vi "test_dragon_file--move_version_to_subtable.vi"(8 "error in (no error)":errorcluster) -> (0 "error out":errorcluster)   [LabVIEW 2020]
uses:
  2bb1123c-6ef6-469c-ba61-7f462a8b3992.vi
  2bb1123c-6ef6-469c-ba61-7f462a8b3992.vi/4178f046-9af6-4db4-9405-99552d650b27.vi
  2bb1123c-6ef6-469c-ba61-7f462a8b3992.vi/504846f3-46c1-483c-ab2c-e4b1da560c38.vi
  toml/write_subtable_key_string.vi
  toml/toml.lvclass
  <vilib>/addons/_JKI Toolkits/Caraya/classes/Assert/Assert.lvclass
  <vilib>/addons/_JKI Toolkits/Caraya/classes/Test/Test.lvclass
panel:
  out "toml_string":string
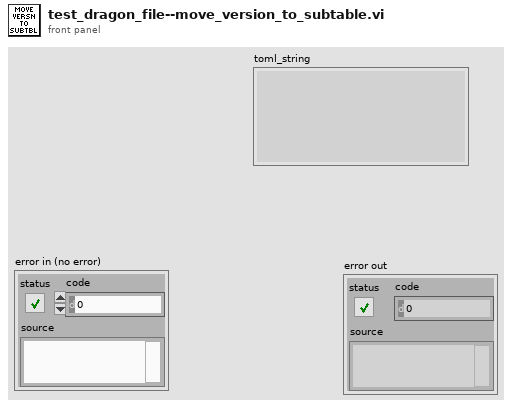
[diagram p1: front panel]
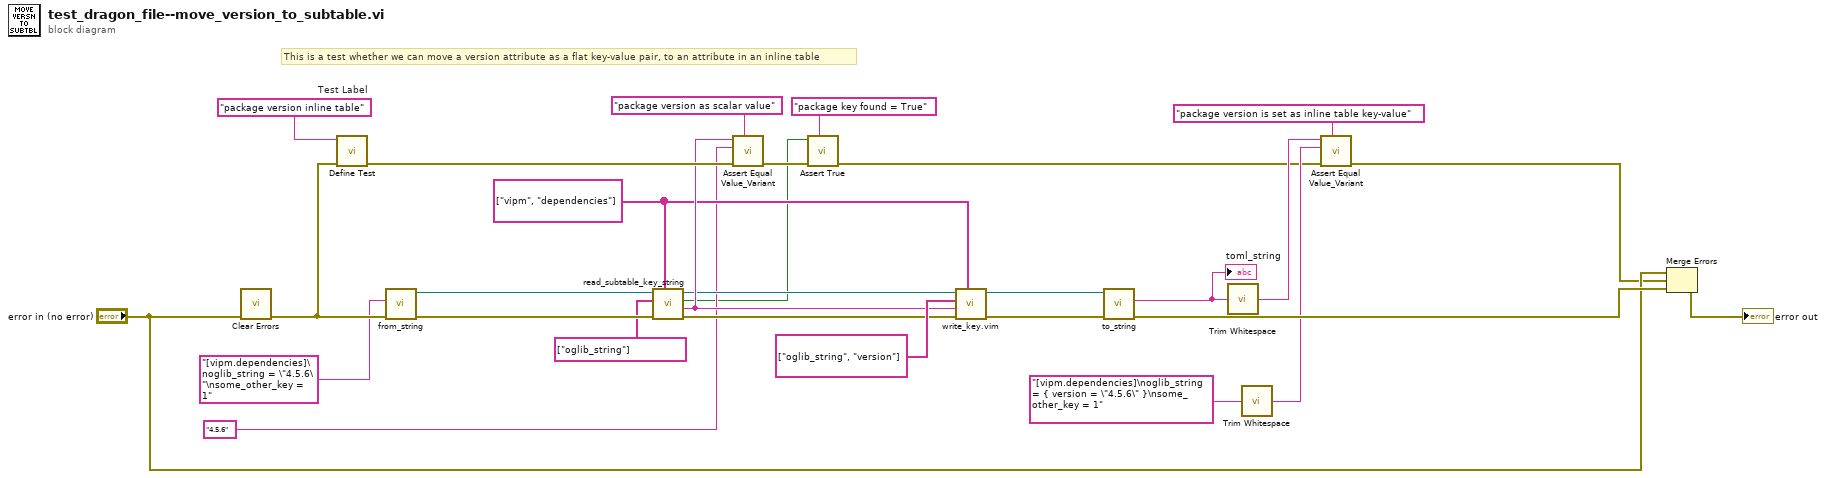
[diagram p0: block diagram]
diagram:
  w16 = string[] ["vipm", "dependencies"]
  w27 = "package version inline table"  # Test Label
  # "This is a test whether we can move a version attribute as a flat key-value pair, to an attribute in an inline table"
  n1 = call <vilib>:"Clear Errors.vi"("error in (no error)"="error in (no error)") -> ("error out"=w14:errorcluster)  [unwired: 5 in, 1 out]
  n2 = call <vilib>:"Define Test.vi"("error in (no error)"=w14, "Label (VI Title)"=w27) -> ("error out"=w28:errorcluster)  [unwired: 9 in]
  n3 = call "from_string.vi"("error in (no error)"=w14, "toml"="[vipm.dependencies]\noglib_string = \"4.5.6\"\nsome_other_key = 1" ("toml_string in")) -> ("error out"=w25:errorcluster, "toml out"=w26:refnum<class "toml.lvclass">)  [unwired: 8 in]
  n4 = call "read_subtable_key_string.vi"("subtables"=w16, "error in (no error)"=w25, "subkeys"=string[] ["oglib_string"], "toml in"=w26) -> ("error out"=w17:errorcluster, "value"=w21:string, "found?"=w3:bool, "toml out"=w18:refnum<class "toml.lvclass">)  [unwired: 4 in]
  n5 = call <vilib>:"Assert Equal Value_Variant.vi"("Label"="package version as scalar value", "error in (no error)"=w28, "Y"="4.5.6" ("table_name"), "X"=w21) -> ("error out"=w4:errorcluster)  [unwired: 7 in]
  n6 = call <vilib>:"Assert True.vi"("Label"="package key found = True", "error in (no error)"=w4, "True?"=w3) -> ("error out"=w1:errorcluster)  [unwired: 8 in]
  n7 = call "write_key.vim"("table"=w16, "error in (no error)"=w17, "value"=w21, "key"=string[] ["oglib_string", "version"], "toml in"=w18) -> ("error out"=w19:errorcluster, "toml out"=w20:refnum<class "toml.lvclass">)  [unwired: 5 in]
  n8 = call "to_string.vi"("error in (no error)"=w19, "toml in"=w20) -> ("error out"=w24:errorcluster, "toml_string"=w11:string)  [unwired: 8 in]
  "toml_string" <- w11
  n9 = call <vilib>:"Trim Whitespace.vi"("string"=w11) -> ("trimmed string"=w10:string)  [unwired: 1 in]
  n10 = call <vilib>:"Trim Whitespace.vi"("string"="[vipm.dependencies]\noglib_string = { version = \"4.5.6\" }\nsome_other_key = 1" ("toml_string in")) -> ("trimmed string"=w8:string)  [unwired: 1 in]
  n11 = call <vilib>:"Assert Equal Value_Variant.vi"("Label"="package version is set as inline table key-value", "error in (no error)"=w1, "Y"=w8, "X"=w10) -> ("error out"=w9:errorcluster)  [unwired: 7 in]
  n12 = Merge Errors("error in (no error)", w9, w24) -> (→"error out":errorcluster)
